vi "Write Array.vi"(8 "error in (no error)":errorcluster, 10 "Array":T1[][](array[typedef]), 11 "Elevator in":refnum<class "Elevator.lvclass">) -> (0 "error out":errorcluster, 3 "Elevator out":refnum<class "Elevator.lvclass">)   [LabVIEW 2018, in "Elevator.lvlib" / "Elevator.lvclass"]
uses:
  Elevator.lvclass
  Controls/Elevator Position.ctl
  Elevator.lvclass/Elevator.ctl
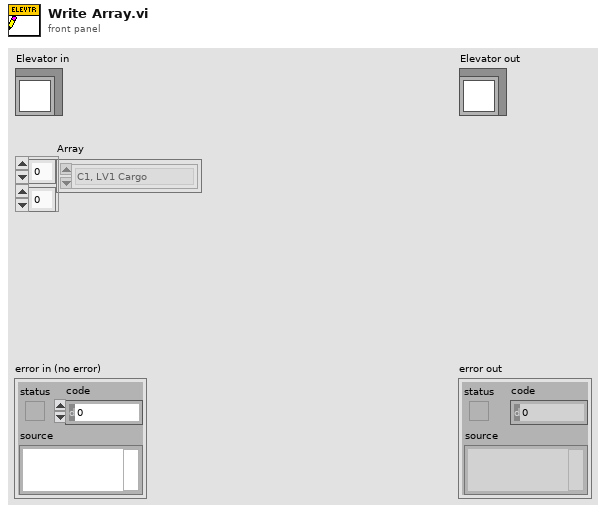
[diagram p1: front panel]
types:
  T1 = typedef "Elevator.lvlib/Elevator.lvclass/Elevator Position.ctl" = enum16{"CS, Cargo Ship Cargo", "C0, Cargo Ground", "C1, LV1 Cargo", "C2, LV2 Cargo", "C3, LV3 Cargo", "H0, LV1 Hatch", "H1, LV2 Hatch", "H2, LV3 Hatch"}
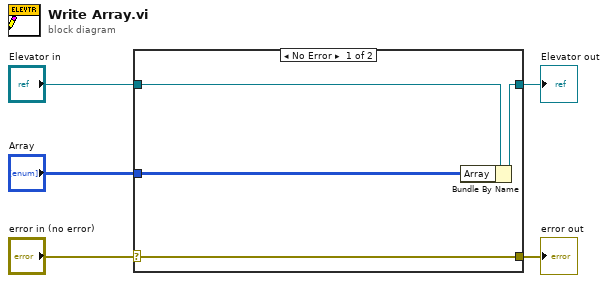
[diagram p0: block diagram]
diagram:
  n1 = case shown="No Error" "error in (no error)" {
    selector: "error in (no error)" -> [w9 w10]
    tunnel: [w9 w10] -> w4
    tunnel: [w7 w11] -> w2
    tunnel: "Elevator in" -> [w8 w11]
    tunnel: "Array" -> [w6 _]
    frame No Error {
      n2 = Bundle By Name(cluster=w8, "Array"=w6) -> (w7:refnum<class "Elevator.lvclass">)
    }
    frame Error {
    }
  }
  "error out" <- w4
  "Elevator out" <- w2
